vi "Sort Mixed Mode Archive Records.vi"(0 "Raw Records":T1[](array[typedef]), 1 "Number of LBCBs":i32) -> (4 "Command Records":string[](array[string]), 5 "Stiffness Records":string[](array[string]))   [LabVIEW 2009]
uses:
  Command or Stiffnness Record.ctl
  Command or Stiffness Updates.ctl
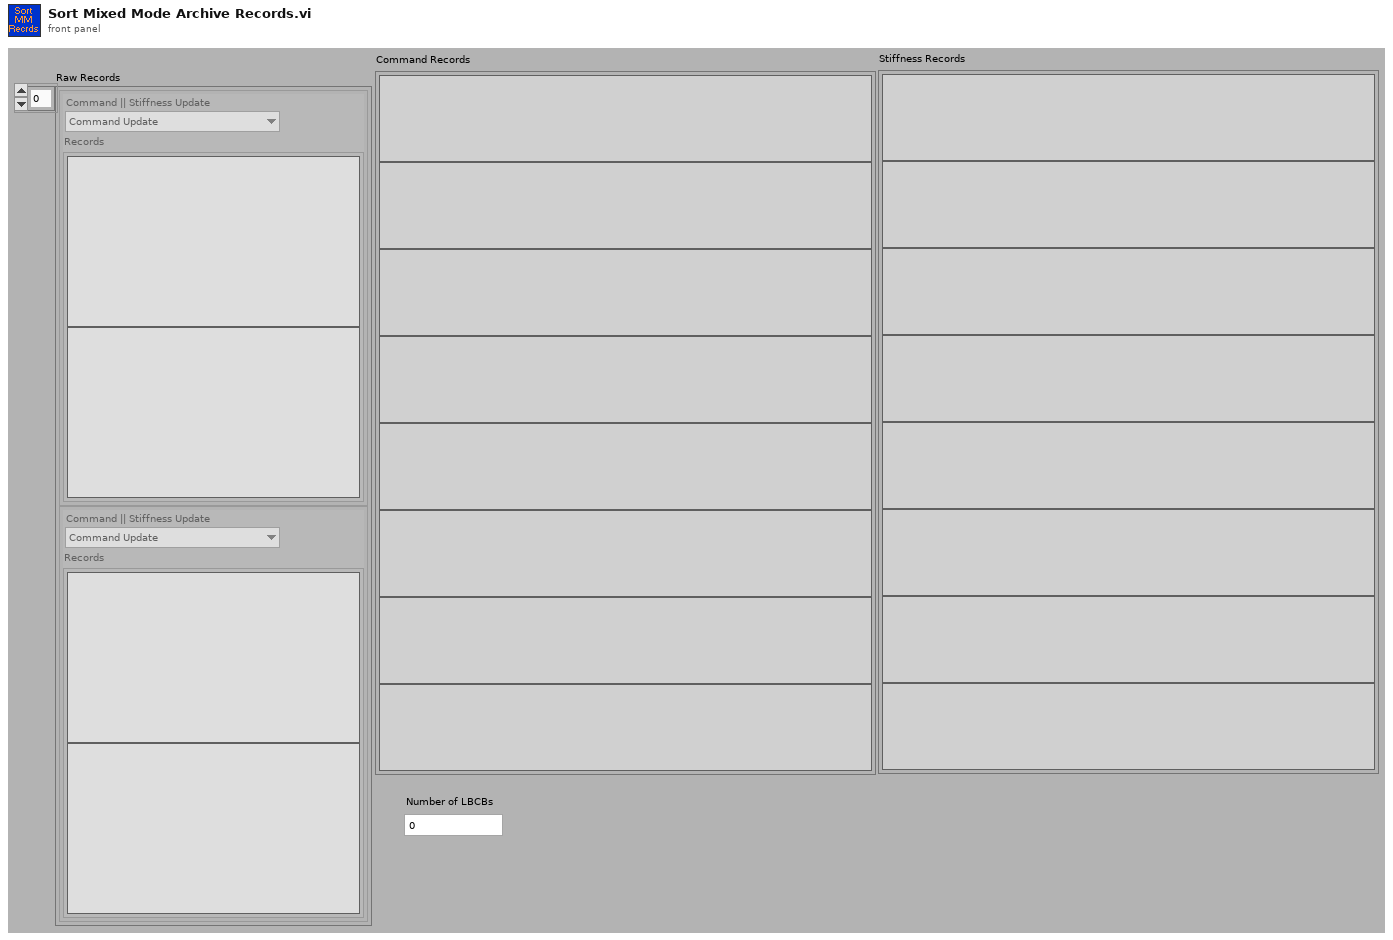
[diagram p1: front panel]
types:
  T1 = typedef "Command or Stiffnness Record.ctl" = cluster{"Command || Stiffness Update":T2, "Records":string[]}
  T2 = typedef "Command or Stiffness Updates.ctl" = enum16{"Command Update", "Iterative Command Update", "Stiffness Update"}
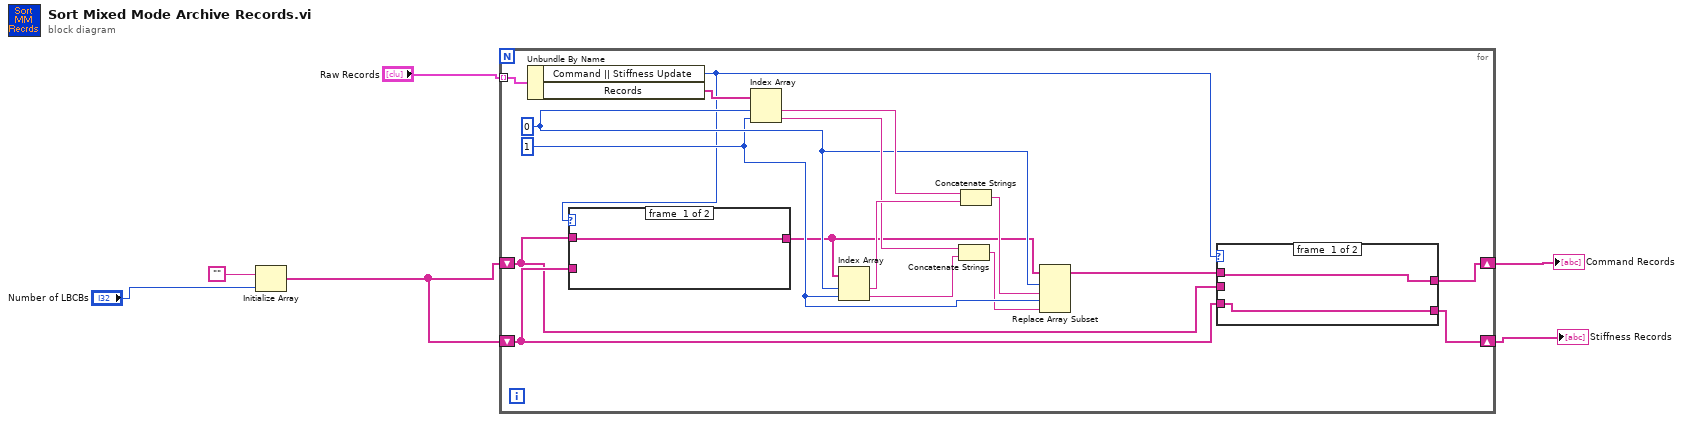
[diagram p0: block diagram]
diagram:
  n1 = Initialize Array("", "Number of LBCBs") -> (w3:string[])
  n2 = for {
    tunnel: "Raw Records" -> [w23] mode=indexing
    shift-right: [w9] -> w4
    shift-left: w3 -> [w7]
    shift-right: [w10] -> w2
    shift-left: w3 -> [w8]
    w16 = 1 ("index")
    w17 = 0 ("index")
    n3 = Unbundle By Name(w23) -> ("Command || Stiffness Update"=w12:T2, "Records"=w22:string[])
    n4 = case shown="\"Stiffness Update\"" w12 {
      tunnel: w7 -> [w28 _]
      tunnel: w8 -> [_ w29]
      tunnel: [w28 w29] -> w13
      frame #0 {
      }
      frame #1 {
      }
    }
    n5 = Index Array(array=w22, index #1=w17, index #2=w16) -> (element #1=w21:string, element #2=w19:string)
    n6 = Index Array(array=w13, index #1=w17, index #2=w16) -> (element #1=w20:string, element #2=w18:string)
    n7 = Concatenate Strings(w19, w18) -> (w14:string)
    n8 = Concatenate Strings(w21, w20) -> (w15:string)
    n9 = Replace Array Subset(array=w13, new element #1=w15, index #1=w17, new element #2=w14, index #2=w16) -> (w11:string[])
    n10 = case shown="\"Stiffness Update\"" w12 {
      tunnel: w11 -> [w25 w27]
      tunnel: [w24 w27] -> w10
      tunnel: [w25 w26] -> w9
      tunnel: w8 -> [w24 _]
      tunnel: w7 -> [_ w26]
      frame #0 {
      }
      frame #1 {
      }
    }
  }
  "Command Records" <- w4
  "Stiffness Records" <- w2
